vi "Configure TIS Mode.vi"(8 "error in":errorcluster, 10 "AI Channel":enum16{"AI 0", "AI 1"}(ring), 11 "FPGA VI Reference In 2":refnum<k20>) -> (0 "error out":errorcluster, 2 "Configuration Error":bool, 3 "FPGA VI Reference Out 2":refnum<k20>)   [LabVIEW 2014]
doc: "This VI configures the Time Interleaved Sampling (TIS) for the NI 5771. For execution steps, refer to the comments on the block diagram."
uses:
  <vilib>/Utility/error.llb/Error Cluster From Error Code.vi
  <vilib>/rvi/errors/niLvFpgaAdjustHostInterfaceError.vi
  <vilib>/rvi/interface/nirviReadWriteControl/nirviReadWriteControl.xnode
  <vilib>/rvi/interface/Simulation/niFpgaSimulationCallBeginRW.vi
  NiFpgaLv.dll
panel:
  # "This VI configures the Time Interleaved Sampling (TIS) for the NI 5771. For execution steps, refer to the comments on the block diagram."
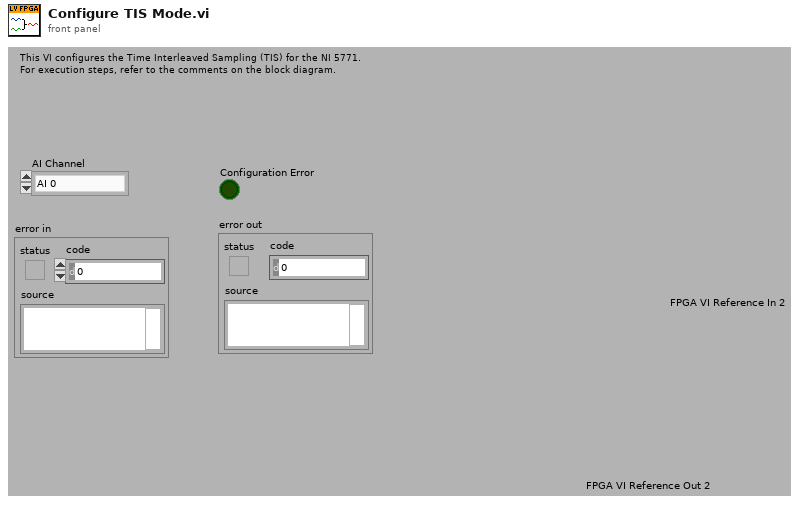
[diagram p1: front panel]
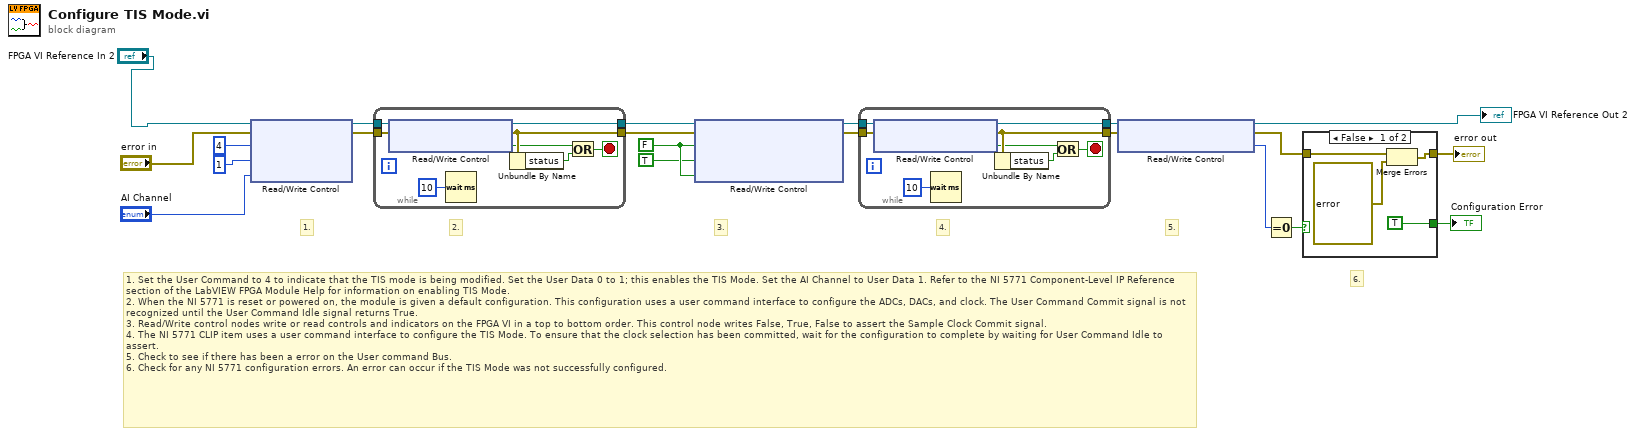
[diagram p0: block diagram]
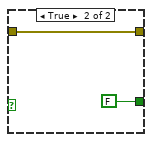
[diagram p2: hidden frame]
diagram:
  w16 = FALSE ("Sample Clock Commit")
  # "5."
  # "1. Set the User Command to 4 to indicate that the TIS mode is being modified. Set the User Data 0 to 1; this enables the TIS Mode. Set the AI Channel to User Data 1. Refer to the NI 5771 Component-Level IP Reference section of the LabVIEW FPGA Module Help for information on enabling TIS Mode.\n2. When the NI 5771 is reset or powered on, the module is given a default configuration. This configuration uses a user command interface to configure the ADCs, DACs, and clock. The User Command Commit signal is not recognized until the User Command Idle signal returns True.\n3. Read/Write control nodes write or read controls and indicators on the FPGA VI in a top to bottom order. This control node writes False, True, False to assert the Sample Clock Commit signal.\n4. The NI 5771 CLIP item uses a user command interface to configure the TIS Mode. To ensure that the clock selection has been committed, wait for the configuration to complete by waiting for User Command Idle to assert.\n5. Check to see if there has been a error on the User command Bus.\n6. Check for any NI 5771 configuration errors. An error can occur if the TIS Mode was not successfully configured."
  # "6."
  # "4."
  # "3."
  # "2."
  # "1."
  n1 = xnode "Read/Write Control"("FPGA VI Reference In"="FPGA VI Reference In 2", "error in"="error in", "User Command"=u8 4, "User Data 0"=u8 1, "User Data 1"="AI Channel") -> ("FPGA VI Reference Out"=w20:refnum<k20>, "error out"=w19:errorcluster)
  n2 = while {
    tunnel: w20 -> [w25]
    tunnel: w19 -> [w26]
    tunnel: [w23] -> w17
    tunnel: [w24] -> w18
    stop <- w27 stop-if-true
    n3 = xnode "Read/Write Control"("FPGA VI Reference In"=w25, "error in"=w26) -> ("FPGA VI Reference Out"=w24:refnum<k20>, "error out"=w23:errorcluster, "User Command Idle"=w22:bool)
    n4 = Wait (ms)(milliseconds to wait=u32 10) -> ()  [unwired: 1 out]
    n5 = Unbundle By Name(w23) -> ("status"=w28:bool)
    n6 = Or(x=w22, y=w28) -> (x .or. y?=w27:bool)
  }
  n7 = xnode "Read/Write Control"("FPGA VI Reference In"=w18, "error in"=w17, "User Command Commit"=w16, "User Command Commit"=TRUE ("Sample Clock Commit"), "User Command Commit"=w16) -> ("FPGA VI Reference Out"=w13:refnum<k20>, "error out"=w12:errorcluster)
  n8 = while {
    tunnel: w13 -> [w33]
    tunnel: w12 -> [w34]
    tunnel: [w31] -> w11
    tunnel: [w32] -> w10
    stop <- w35 stop-if-true
    n9 = xnode "Read/Write Control"("FPGA VI Reference In"=w33, "error in"=w34) -> ("FPGA VI Reference Out"=w32:refnum<k20>, "error out"=w31:errorcluster, "User Command Idle"=w30:bool)
    n10 = Wait (ms)(milliseconds to wait=u32 10) -> ()  [unwired: 1 out]
    n11 = Unbundle By Name(w31) -> ("status"=w36:bool)
    n12 = Or(x=w30, y=w36) -> (x .or. y?=w35:bool)
  }
  n13 = xnode "Read/Write Control"("FPGA VI Reference In"=w10, "error in"=w11) -> ("FPGA VI Reference Out"=→"FPGA VI Reference Out 2":refnum<k20>, "error out"=w8:errorcluster, "User Command Status"=w6:u8)
  n14 = Equal To 0?(x=w6) -> (x = 0?=w5:bool)
  n15 = case shown="False" w5 {
    tunnel: [w41 w43] -> w14
    tunnel: w8 -> [w40 w43]
    tunnel: [TRUE ("Configured?") FALSE ("Configured?")] -> w7
    frame False {
      n16 = Merge Errors(w40, errorcluster {"status"=TRUE, "code"=-8998, "source"="IO Module clock not configured correctly. Please ensure that the desired clock meets the required specifications."} ("error in")) -> (w41:errorcluster)
    }
    frame True {
    }
  }
  "error out" <- w14
  "Configuration Error" <- w7
